vi "FT10_Semi-Auto Read and Wait.vi"(8 "Activation Duration":T4, 9 "Mode in":T2, 10 "Port in":T3, 11 "Read Frequency":i32) -> (1 "Mode out":T2, 2 "Port out":T3, 3 "Command Cluster Array":T1[](array[typedef]))   [LabVIEW 2024]
doc: "Creates message for Message Handling Loop to read current & voltage at specified frequency (ms) and wait between reads."
uses:
  Controls/Control_Semi-Auto Activation Duration.ctl
  Controls/Control_Semi-Auto Port.ctl
  Controls/Control_Semi-Auto Mode.ctl
  Controls/Control_Command Cluster.ctl
  Controls/Control_M4X Read Current Bool.ctl
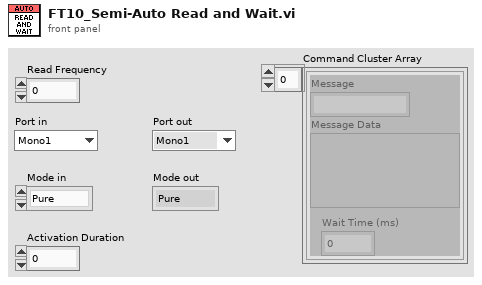
[diagram p1: front panel]
types:
  T1 = typedef "Control_Command Cluster.ctl" = cluster{"Message":string, "Message Data":variant, "Wait Time (ms)":i32}
  T2 = typedef "Control_Semi-Auto Mode.ctl" = enum16{"Pure", "Blend", "Spray", "Fulgerate", "Standard", "Macro", "Precision", "Ligasure", "Error"}
  T3 = typedef "Control_Semi-Auto Port.ctl" = enum16{"Mono1", "Mono2", "Bipolar", "Ligasure", "Error"}
  T4 = typedef "Control_Semi-Auto Activation Duration.ctl" = i32
  T5 = typedef "Control_M4X Read Current Bool.ctl" = bool
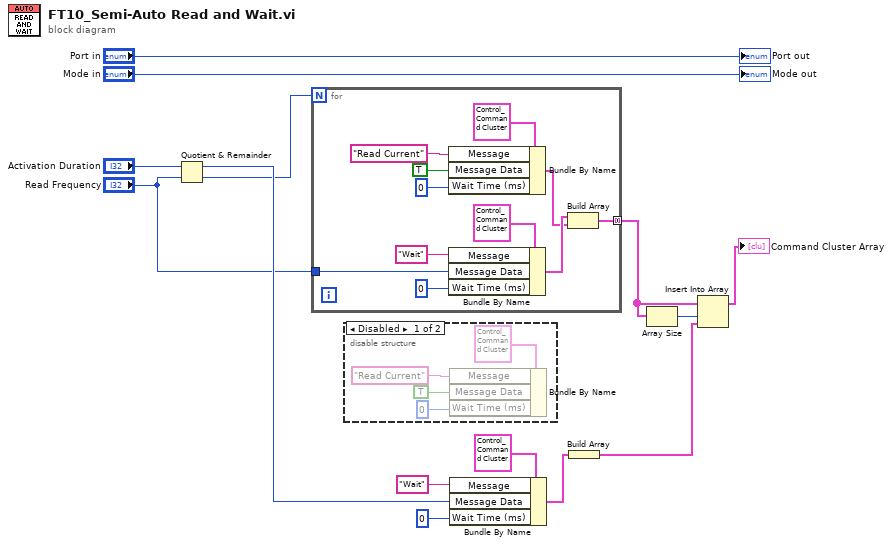
[diagram p0: block diagram]
diagram:
  n1 = Quotient & Remainder(x="Activation Duration", y="Read Frequency") -> (x-y*floor(x/y)=w12:T4, floor(x/y)=w7:T4)
  n2 = for {
    N: w7 -> [_]
    tunnel: "Read Frequency" -> [w18]
    tunnel: [w17] -> w4 mode=concatenating
    n3 = Bundle By Name(cluster=T1 {"Message"="", "Message Data"=variant, "Wait Time (ms)"=0}, "Message"="Read Current", "Message Data"=T5 TRUE ("Read Current"), "Wait Time (ms)"=0) -> (w15:T1)
    n4 = Bundle By Name(cluster=T1 {"Message"="", "Message Data"=variant, "Wait Time (ms)"=0}, "Message"="Wait", "Message Data"=w18, "Wait Time (ms)"=0) -> (w16:T1)
    n5 = Build Array(w16, w15) -> (w17:T1[])
  }
  n6 = disable-structure shown="Disabled" {
    frame Disabled {
      n7 = Bundle By Name(cluster=T1 {"Message"="", "Message Data"=variant, "Wait Time (ms)"=0}, "Message"="Read Current", "Message Data"=T5 TRUE ("Read Current 2"), "Wait Time (ms)"=0) -> ()  [unwired: 1 out]
    }
    frame Enabled {
    }
  }
  n8 = Bundle By Name(cluster=T1 {"Message"="", "Message Data"=variant, "Wait Time (ms)"=0}, "Message"="Wait", "Message Data"=w12, "Wait Time (ms)"=0) -> (w11:T1)
  n9 = Build Array(w11) -> (w2:T1[])
  n10 = Array Size(array=w4) -> (size(s)=w3:i32)
  n11 = Insert Into Array(array=w4, index=w3, new element=w2) -> (→"Command Cluster Array":T1[])
  "Port out" <- "Port in"
  "Mode out" <- "Mode in"
